vi "ParaDelete.vi"(11 "段名":string) -> ()   [LabVIEW 2018]
uses:
  <vilib>/Utility/config.llb/NI_LVConfig.lvlib
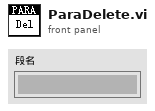
[diagram p1: front panel]
types:
  T1 = typedef "NI_LVConfig.lvlib/Config Data RefNum.ctl" = refnum<k1>
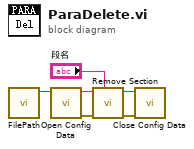
[diagram p0: block diagram]
diagram:
  n1 = call "FilePath.vi"() -> ("添加的路径"=w6:path)  [unwired: 11 in]
  n2 = call <vilib>:"Open Config Data.vi"("configuration file path"=w6) -> ("error out"=w3:errorcluster, "refnum"=w5:T1)  [unwired: 8 in, 1 out]
  n3 = call <vilib>:"Remove Section.vi"("section"="段名", "error in (no error)"=w3, "refnum"=w5) -> ("error out"=w1:errorcluster, "refnum out"=w2:T1)  [unwired: 6 in, 1 out]
  n4 = call <vilib>:"Close Config Data.vi"("error in (no error)"=w1, "refnum"=w2) -> ()  [unwired: 8 in, 2 out]
